vi "Medidor.vi"() -> ()   [LabVIEW 2020]
panel:
  out "Lectura":string
  out "Medidor":dbl(knob) scale=0.0..10.0
  in  "Apagar Medidor":bool
  in  "Selector":u16(ring) items=["Corriente", "Resistencia", "Voltaje"]
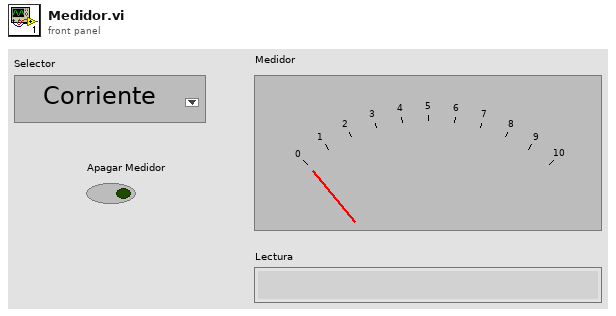
[diagram p1: front panel]
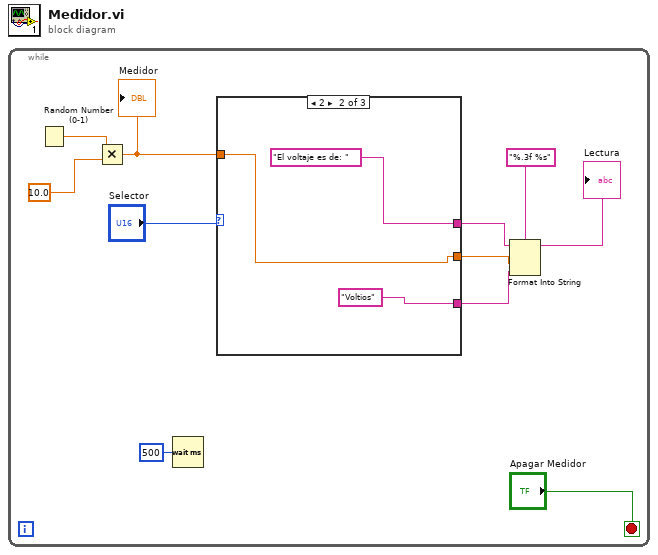
[diagram p0: block diagram]
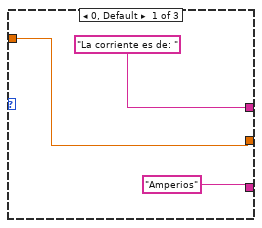
[diagram p2: hidden frame]
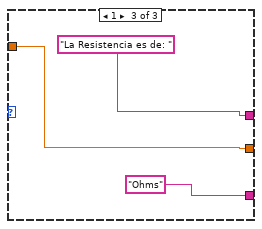
[diagram p3: hidden frame]
diagram:
  n1 = while {
    stop <- "Apagar Medidor" stop-if-true
    n2 = Random Number (0-1)() -> (number: 0 to 1=w8:dbl)
    n3 = Multiply(x=w8, y=10.0) -> (x*y=w7:dbl)
    "Medidor" <- w7
    n4 = Wait (ms)(milliseconds to wait=u32 500) -> ()  [unwired: 1 out]
    n5 = case shown="2" "Selector" {
      tunnel: w7 -> [w13 w17 w19]
      tunnel: ["La corriente es de: " "El voltaje es de: " "La Resistencia es de: "] -> w6
      tunnel: [w13 w17 w19] -> w5
      tunnel: ["Amperios" "Voltios" "Ohms"] -> w4
      frame 0, Default {
      }
      frame 2 {
      }
      frame 1 {
      }
    }
    n6 = Format Into String(format string="%.3f %s", initial string=w6, w5, w4) -> (resulting string=→"Lectura":string)  [unwired: 1 in, 1 out]
  }
